vi "Hybrid tesla2kA.vi"(2 "Magnet Field [T]":dbl=1.0 format="%.4f") -> (0 "Current [kA]":dbl=1.0 format="%.4f")   [LabVIEW 2024]
uses:
  PS Comm Globals.vi
panel:
  in  "SC Current [kA]":dbl format="%.5f"
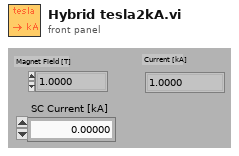
[diagram p1: front panel]
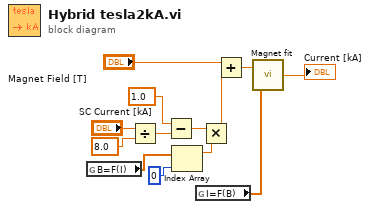
[diagram p0: block diagram]
diagram:
  n1 = global read "PS Comm Globals.vi" "B=F(I)"() -> (w1:dbl[])
  n2 = Divide(x="SC Current [kA]", y=8.0) -> (x/y=w8:dbl)
  n3 = Subtract(x=1.0, y=w8) -> (x-y=w6:dbl)
  n4 = Index Array(array=w1, index=0) -> (element=w5:dbl)
  n5 = global read "PS Comm Globals.vi" "I=F(B)"() -> (w2:dbl[])
  n6 = Multiply(x=w6, y=w5) -> (x*y=w3:dbl)
  n7 = Add(x="Magnet Field [T]", y=w3) -> (x+y=w12:dbl)
  n8 = call "Magnet fit.vi"("Coefficients"=w2, "Magnet Parameter"=w12) -> ("Conjugate Parameter"=→"Current [kA]":dbl)
